vi "ex_WriteDataAll.vi"(0 "file path":path, 1 "File refnum in":refnum<file>, 2 "Signals":waveform(dbl)[](array[waveform]), 3 "overwrite_mode_multi":T3(ring)=enum."overwrite & backup", 4 "overwrite_mode":T4(ring)=enum."overwrite & backup", 5 "error in (no error)":errorcluster, 6 "file dialog?":bool, 7 "Description":string, 8 "multi_file":bool, 9 "Comment":string, 10 "new file?":bool, 11 "Simulate Non-First Call":bool, 12 "file params":T1={"delimiter"="\t", "origin time"=timestamp(0 s since 1904-01-01), "Flags"={"include col headings?"=TRUE, "x_columns"=0, "col headings always?"=TRUE, "time preference"=0, "hide col headings"=FALSE}, "Decimal Separator"=""} {"Flags"."time preference" items=["Absolute", "Relative"]; "Flags"."x_columns" items=["None", "One", "Multiple"]; "origin time" format="%<%X\n%x>T"}) -> (13 "operator cancelled?":bool, 14 "file path out":path, 15 "refnum out":refnum<file>, 17 "mark after write (bytes)":i32, 19 "error out":errorcluster)   [LabVIEW 2017]
uses:
  <vilib>/express/express output/ExFileWriteBlock.llb/ex_WriteFileParams.ctl
  <vilib>/express/express input/ExFileReadBlock.llb/ex_ReadFileParams.ctl
  <vilib>/express/express shared/ExFile.llb/ex_FileGlobals.vi
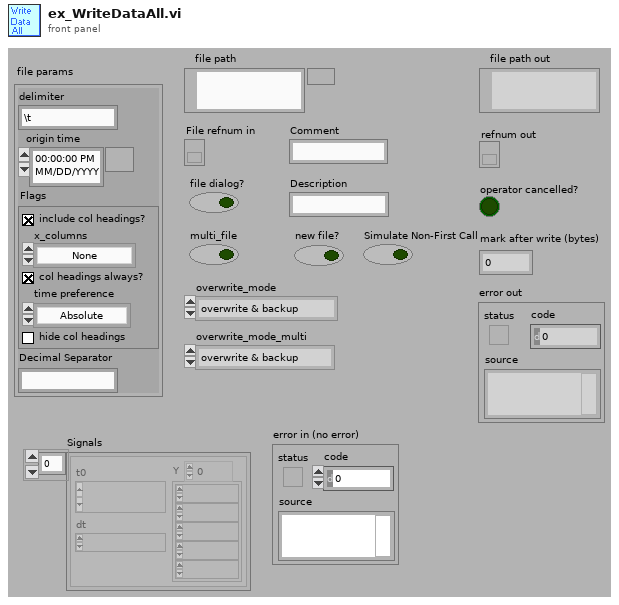
[diagram p1: front panel]
types:
  T1 = typedef "ex_WriteFileParams.ctl" = cluster{"delimiter":string, "origin time":timestamp, "Flags":T2, "Decimal Separator":string}
  T2 = typedef "ex_ReadFileParams.ctl" = cluster{"include col headings?":bool, "x_columns":u16, "col headings always?":bool, "time preference":u16, "hide col headings":bool}
  T3 = enum16{"overwrite", "overwrite & backup", "next avail"}
  T4 = enum16{"overwrite", "overwrite & backup", "append", "next avail"}
  T5 = enum16{"open", "open or create", "create or replace", "create", "open (read only)"}
  T6 = enum16{"existing file", "new file", "new or existing file", "existing dir", "new dir", "new or existing dir", "existing file (use LLBs)", "new file (use LLBs)", "new or existing file (use LLBs)", "new or existing file or directory (use LLBs)"}
  T7 = cluster{"message":string, "T button name":string, "F button name":string}
  T8 = cluster{"Start Timestamp":timestamp, "Timestamp":timestamp, "Relative Time?":bool, "X Dimension":string, "Signal Name":string, "Y Units":string, "X0":timestamp, "dX":dbl, "nPoints":i32}[]
  T9 = typedef "ex_WaveformAttribsPlus.ctl" = cluster{"Start Timestamp":timestamp, "Timestamp":timestamp, "Relative Time?":bool, "X Dimension":string, "Signal Name":string, "Y Units":string, "X0":timestamp, "dX":dbl, "nPoints":i32}
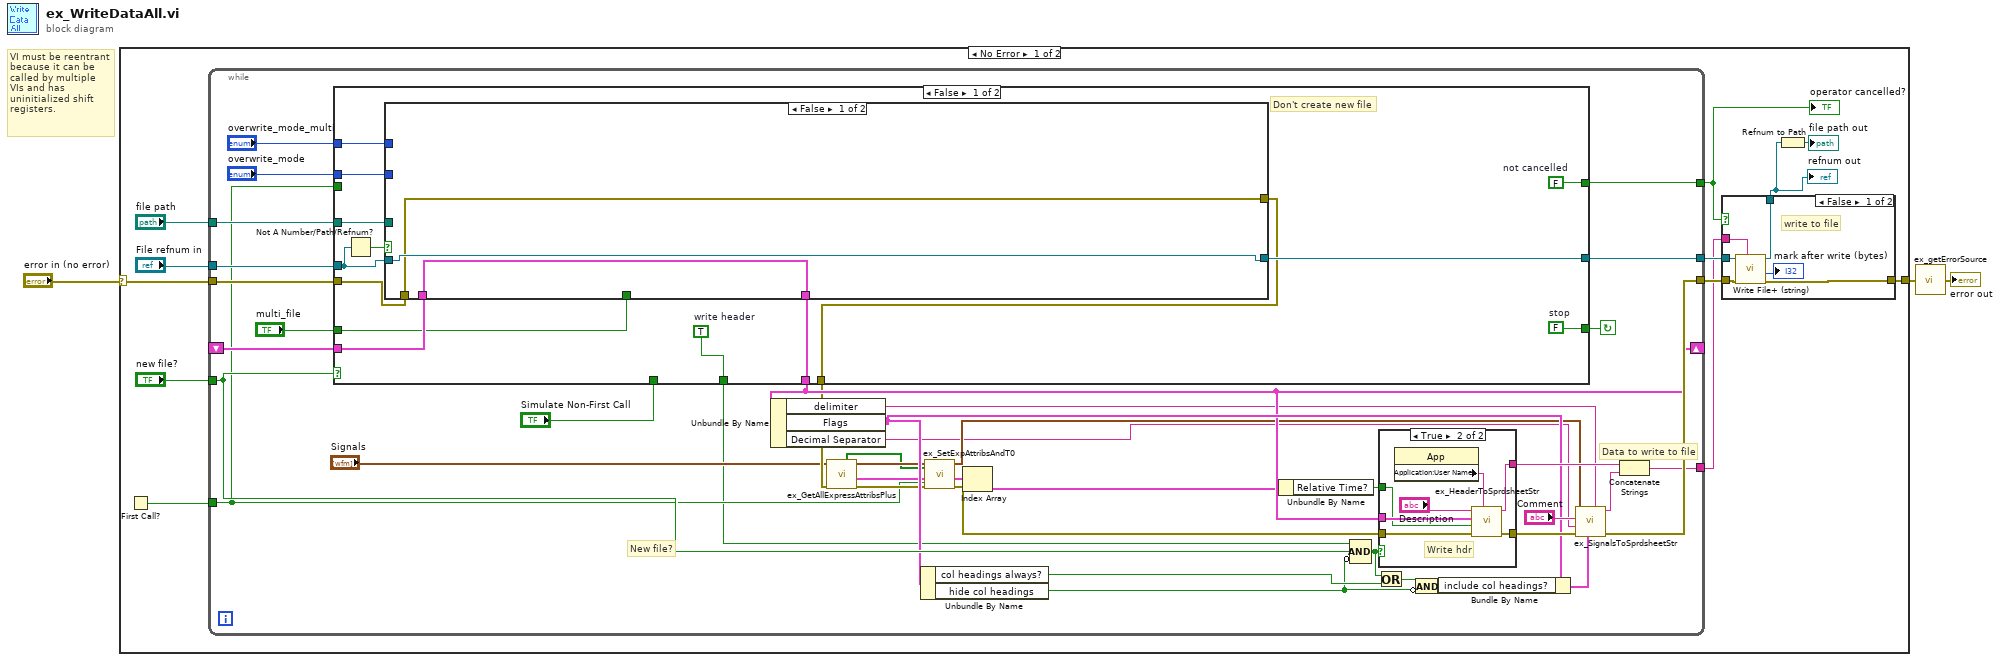
[diagram p0: block diagram]
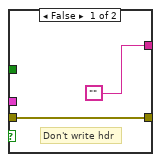
[diagram p2: hidden frame]
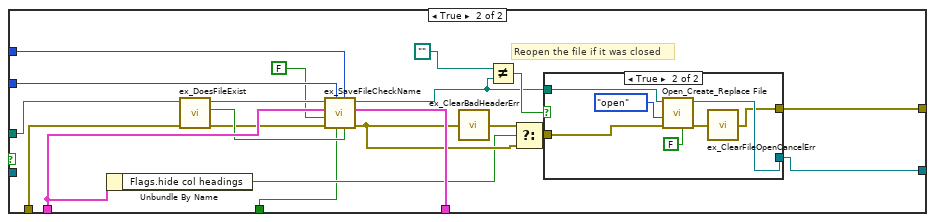
[diagram p3: hidden frame]
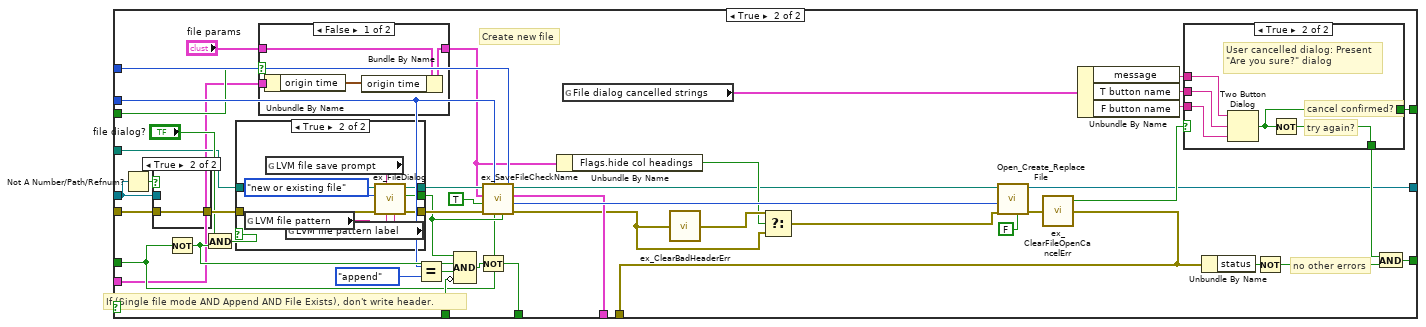
[diagram p5: hidden frame]
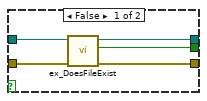
[diagram p8: hidden frame]
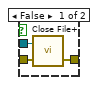
[diagram p9: hidden frame]
diagram:
  # "VI must be reentrant\nbecause it can be\ncalled by multiple\nVIs and has\nuninitialized shift\nregisters."
  n1 = case shown="No Error" "error in (no error)" {
    selector: "error in (no error)" -> [w15 w193]
    tunnel: [w12 w193] -> w2
    frame No Error {
      n2 = First Call?() -> (First Call?: T/F=w7:bool)
      n3 = while {
        tunnel: w15 -> [w56]
        tunnel: "File refnum in" -> [w55]
        tunnel: "new file?" -> [w48]
        tunnel: [w50] -> w11
        tunnel: [w43] -> w10
        tunnel: [w44] -> w9
        tunnel: "file path" -> [w54]
        tunnel: [w49] -> w8
        shift-right: [w39] -> _
        shift-left: _ -> [w41]
        tunnel: w7 -> [w19]
        stop <- w45 continue-if-true
        # "New file?"
        # "Data to write to file"
        n4 = case shown="False" w48 {
          tunnel: w56 -> [w71 w153]
          tunnel: w55 -> [w75 w154]
          tunnel: w54 -> [w73 w128]
          tunnel: [w72 w137] -> w34
          tunnel: [w79 w142] -> w45
          tunnel: [w78 w136] -> w44
          tunnel: [w68 w134] -> w39
          tunnel: [w74 w135] -> w43
          tunnel: w41 -> [w69 w114]
          tunnel: [w77 w129] -> w18
          tunnel: "Simulate Non-First Call" -> [_ w121]
          tunnel: "overwrite_mode_multi" -> [w67 w120]
          tunnel: "overwrite_mode" -> [w70 w119]
          tunnel: "multi_file" -> [w66 w118]
          tunnel: w19 -> [_ w115]
          frame False {
            w77 = TRUE  # write header
            w78 = FALSE  # not cancelled
            w79 = FALSE  # stop
            # "Don't create new file"
            n5 = Not A Number/Path/Refnum?(number/path/refnum=w75) -> (NaN/Path/Refnum?=w76:bool)
            n6 = case shown="False" w76 {
              tunnel: w75 -> [w82 _]
              tunnel: [w82 w99] -> w74
              tunnel: w73 -> [_ w91]
              tunnel: w71 -> [w81 w89]
              tunnel: [w81 w98] -> w72
              tunnel: w70 -> [_ w101]
              tunnel: w69 -> [w80 w95]
              tunnel: [w80 w102] -> w68
              tunnel: w67 -> [_ w100]
              tunnel: w66 -> [_ w87]
              frame False {
              }
              frame True {
                # "Reopen the file if it was closed"
                n7 = Unbundle By Name(w95) -> ("Flags.hide col headings"=w94:bool)
                n8 = call <vilib>:"ex_DoesFileExist.vi"("error in"=w89, "file path"=w91) -> ("error out"=w88:errorcluster, "file exists"=w92:bool, "dup file path"=w90:path)  [unwired: 3 out]
                n9 = call <vilib>:"ex_SaveFileCheckName.vi"("file exists?"=w92, "overwrite_mode_multi"=w100, "multi_file"=w87, "overwrite_mode"=w101, "error in (no error)"=w88, "enable file ops"=FALSE, "file params in"=w95, "file path"=w90) -> ("error out"=w96:errorcluster, "file params out"=w102:T1, "file path out"=w83:path)  [unwired: 1 out]
                n10 = call <vilib>:"ex_ClearBadHeaderErr.vi"("error in"=w96) -> ("error out"=w97:errorcluster)  [unwired: 4 out]
                n11 = Not Equal?(x=path "", y=w83) -> (x != y?=w85:bool)
                n12 = Select(t=w97, s=w94, f=w96) -> (s? t:f=w93:errorcluster)
                n13 = case shown="True" w85 {
                  tunnel: w83 -> [_ w107]
                  tunnel: [_ w106] -> w99
                  tunnel: [w103 w105] -> w98
                  tunnel: w93 -> [w103 w104]
                  frame False {
                  }
                  frame True {
                    n14 = call <vilib>:"Open_Create_Replace File.vi"("advisory dialog? (display:T)"=FALSE, "error in (no error)"=w104, "function (open:0)"=T5."open", "file path"=w107) -> ("error out"=w109:errorcluster, "refnum"=w106:refnum<file>)  [unwired: 3 in, 3 out]
                    n15 = call <vilib>:"ex_ClearFileOpenCancelErr.vi"("error in"=w109) -> ("error out"=w105:errorcluster)  [unwired: 4 out]
                  }
                }
              }
            }
          }
          frame True {
            # "If (Single file mode AND Append AND File Exists), don't write header."
            # "no other errors"
            # "Create new file"
            n16 = Not A Number/Path/Refnum?(number/path/refnum=w154) -> (NaN/Path/Refnum?=w155:bool)
            n17 = case shown="True" w155 {
              tunnel: [w183 w184] -> w151
              tunnel: w153 -> [w182 w184]
              tunnel: w154 -> [w181 _]
              frame False {
                n18 = call <vilib>:"Close File+.vi"("error in (no error)"=w182, "refnum"=w181) -> ("error out"=w183:errorcluster)  [unwired: 5 out]
              }
              frame True {
              }
            }
            n19 = Not(x=w118) -> (.not. x?=w149:bool)
            n20 = And(x="file dialog?", y=w149) -> (x .and. y?=w148:bool)
            n21 = case shown="True" w148 {
              tunnel: w128 -> [w170 w180]
              tunnel: [w169 w179] -> w133
              tunnel: [w168 w178] -> w152
              tunnel: w151 -> [w171 w177]
              tunnel: [w167 w176] -> w130
              frame False {
                n22 = call <vilib>:"ex_DoesFileExist.vi"("error in"=w171, "file path"=w170) -> ("error out"=w168:errorcluster, "file exists"=w167:bool, "dup file path"=w169:path)  [unwired: 3 out]
              }
              frame True {
                n23 = global read "ex_FileGlobals.vi" "LVM file pattern"() -> (w172:string)
                n24 = global read "ex_FileGlobals.vi" "LVM file save prompt"() -> (w174:string)
                n25 = global read "ex_FileGlobals.vi" "LVM file pattern label"() -> (w173:string)
                n26 = call <vilib>:"ex_FileDialog.vi"("pattern label"=w173, "pattern"=w172, "prompt"=w174, "error in (no error)"=w177, "select mode"=T6."new or existing file", "start path"=w180) -> ("error out"=w178:errorcluster, "file exists?"=w176:bool, "selected file path"=w179:path)  [unwired: 3 out]
              }
            }
            n27 = case shown="False" w115 {
              tunnel: "file params" -> [w159 w160]
              tunnel: [w158 w160] -> w111
              tunnel: w114 -> [w157 _]
              frame False {
                n28 = Unbundle By Name(w157) -> ("origin time"=w156:timestamp)
                n29 = Bundle By Name(cluster=w159, "origin time"=w156) -> (w158:T1)
              }
              frame True {
              }
            }
            n30 = Equal?(x=w119, y=T4."append" ("overwrite_mode")) -> (x = y?=w131:bool)
            n31 = Compound Arithmetic op=AND(w130, w149, w131, invert w121) -> (w113:bool)
            n32 = Not(x=w113) -> (.not. x?=w129:bool)
            n33 = call <vilib>:"ex_SaveFileCheckName.vi"("file exists?"=w130, "overwrite_mode_multi"=w120, "multi_file"=w118, "overwrite_mode"=w119, "error in (no error)"=w152, "enable file ops"=TRUE, "file params in"=w111, "file path"=w133) -> ("error out"=w124:errorcluster, "function"=w141:T5, "file params out"=w134:T1, "file path out"=w112:path)
            n34 = Unbundle By Name(w111) -> ("Flags.hide col headings"=w123:bool)
            n35 = global read "ex_FileGlobals.vi" "File dialog cancelled strings"() -> (w127:T7)
            n36 = call <vilib>:"ex_ClearBadHeaderErr.vi"("error in"=w124) -> ("error out"=w125:errorcluster)  [unwired: 4 out]
            n37 = Select(t=w125, s=w123, f=w124) -> (s? t:f=w126:errorcluster)
            n38 = call <vilib>:"Open_Create_Replace File.vi"("advisory dialog? (display:T)"=FALSE, "error in (no error)"=w126, "function (open:0)"=w141, "file path"=w112) -> ("error out"=w122:errorcluster, "refnum"=w135:refnum<file>)  [unwired: 3 in, 3 out]
            n39 = call <vilib>:"ex_ClearFileOpenCancelErr.vi"("error in"=w122) -> ("error out"=w137:errorcluster, "cancelled?"=w147:bool)  [unwired: 3 out]
            n40 = Unbundle By Name(w127) -> ("message"=w140:string, "T button name"=w139:string, "F button name"=w138:string)
            n41 = case shown="True" w147 {
              selector: w147 -> [w161 _]
              tunnel: [w161 w165] -> w144
              tunnel: [w161 w166] -> w136
              tunnel: w138 -> [_ w164]
              tunnel: w140 -> [_ w163]
              tunnel: w139 -> [_ w162]
              frame False {
                # "not cancelled"
                # "file dialog not cancelled"
              }
              frame True {
                # "cancel confirmed?"
                # "try again?"
                # "User cancelled dialog: Present\n\"Are you sure?\" dialog"
                n42 = Two Button Dialog(message=w163, 1:w164, 2:w162) -> (T button?=w166:bool)
                n43 = Not(x=w166) -> (.not. x?=w165:bool)
              }
            }
            n44 = Unbundle By Name(w137) -> ("status"=w145:bool)
            n45 = Not(x=w145) -> (.not. x?=w143:bool)
            n46 = And(x=w144, y=w143) -> (x .and. y?=w142:bool)
          }
        }
        n47 = Unbundle By Name(w39) -> ("delimiter"=w37:string, "Flags"=w42:T2, "Decimal Separator"=w16:string)
        n48 = call <vilib>:"ex_GetAllExpressAttribsPlus.vi"("error in"=w34, "Signals in"="Signals") -> ("error out"=w33:errorcluster, "All Express Wave Attributes Plus"=w32:T8, "Signals out"=w31:waveform(dbl)[], "Time Attribs Not Found"=w29:bool[])  [unwired: 6 out]
        n49 = Unbundle By Name(w42) -> ("col headings always?"=w38:bool, "hide col headings"=w27:bool)
        n50 = call <vilib>:"ex_SetExpAttribsAndT0.vi"("Latch Origin TS? (T)"=w19, "Set? (T if empty)"=w29, "error in (no error)"=w33, "Express Attributes Plus in"=w32, "Signals"=w31) -> ("error out"=w17:errorcluster, "Express Wave Attributes Plus out"=w30:T9[], "Signals With Attributes"=w24:waveform(dbl)[])  [unwired: 1 in, 3 out]
        n51 = Index Array(array=w30) -> (element=w36:T9)  [unwired: 1 in]
        n52 = Unbundle By Name(w36) -> ("Relative Time?"=w35:bool)
        n53 = Compound Arithmetic op=AND(w18, w48, invert w27) -> (w25:bool)
        n54 = Or(x=w25, y=w38) -> (x .or. y?=w40:bool)
        n55 = case shown="True" w25 {
          tunnel: ["" w65] -> w47
          tunnel: [w57 w64] -> w52
          tunnel: w17 -> [w57 w63]
          tunnel: w39 -> [_ w61]
          tunnel: w35 -> [_ w60]
          frame False {
            # "Don't write hdr"
          }
          frame True {
            # "Write hdr"
            n56 = property class="App"() -> ("Application:User Name"=w59:string)  [unwired: 2 in, 2 out]
            n57 = call <vilib>:"ex_HeaderToSprdsheetStr.vi"("operator name"=w59, "error in (no error)"=w63, "Relative Time?"=w60, "file params in"=w61, "description"="Description") -> ("error out"=w64:errorcluster, "spreadsheet string"=w65:string)  [unwired: 1 in, 4 out]
          }
        }
        n58 = Compound Arithmetic op=AND(w40, invert w27) -> (w28:bool)
        n59 = Bundle By Name(cluster=w42, "include col headings?"=w28) -> (w51:T2)
        n60 = call <vilib>:"ex_SignalsToSprdsheetStr.vi"("delimiter (Tab)"=w37, "Flags"=w51, "error in (no error)"=w52, "Decimal Separator"=w16, "comment"="Comment", "Signals"=w24) -> ("error out"=w50:errorcluster, "spreadsheet string"=w53:string)  [unwired: 4 out]
        n61 = Concatenate Strings(w47, w53) -> (w49:string)
      }
      "operator cancelled?" <- w9
      n62 = case shown="False" w9 {
        tunnel: w8 -> [w185 _]
        tunnel: [w189 w191] -> w12
        tunnel: w11 -> [w188 w191]
        tunnel: w10 -> [w187 w192]
        tunnel: [w186 w192] -> w4
        frame False {
          # "write to file"
          n63 = call <vilib>:"Write File+ (string).vi"("string"=w185, "error in (no error)"=w188, "refnum"=w187) -> ("error out"=w189:errorcluster, "mark after write (bytes)"=→"mark after write (bytes)":i32, "dup refnum"=w186:refnum<file>)  [unwired: 2 in, 2 out]
        }
        frame True {
          # "don't write to file"
        }
      }
      "refnum out" <- w4
      n64 = Refnum to Path(1:w4) -> (0:→"file path out":path)
    }
    frame Error {
    }
  }
  n65 = call <vilib>:"ex_getErrorSource.vi"("error in (no error)"=w2) -> ("error out"=→"error out":errorcluster)
